vi "ini Read Key.vi"(0 "Refnum in":T1, 1 "Section":string, 2 "Key":string, 5 "Error In":errorcluster) -> (14 "Refnum out":T1, 15 "value":string, 19 "error out":errorcluster)   [LabVIEW 2016, in "Application.lvclass"]
uses:
  Application.lvclass
  <vilib>/Utility/config.llb/Config Data RefNum.ctl
  <vilib>/Utility/config.llb/Read Key (String).vi
  <vilib>/Utility/config.llb/NI_LVConfig.lvlib
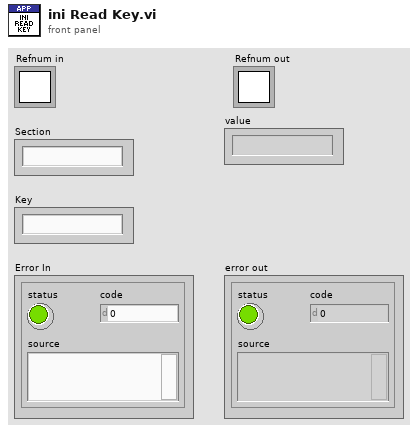
[diagram p1: front panel]
types:
  T1 = typedef "NI_LVConfig.lvlib/Config Data RefNum.ctl" = refnum<k1>
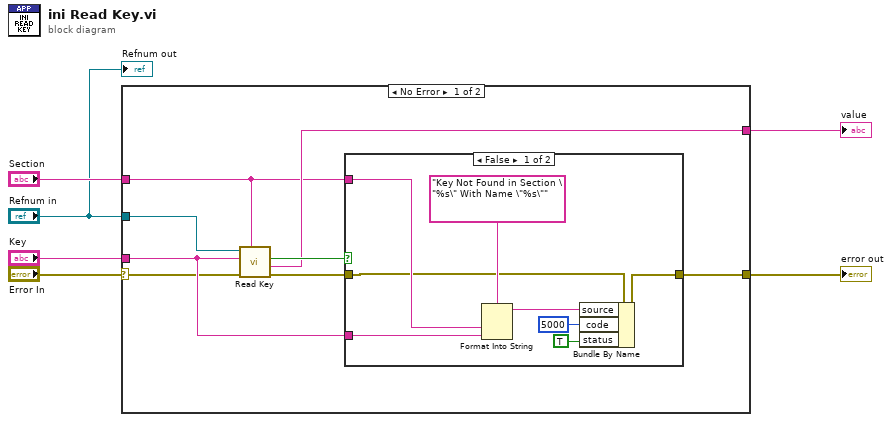
[diagram p0: block diagram]
diagram:
  n1 = case shown="No Error" "Error In" {
    selector: "Error In" -> [w7 w24]
    tunnel: [w14 w24] -> w6
    tunnel: [w11 _] -> w5
    tunnel: "Refnum in" -> [w10 _]
    tunnel: "Key" -> [w9 _]
    tunnel: "Section" -> [w8 _]
    frame No Error {
      n2 = call-poly <vilib>:"Read Key.vi"("section"=w8, "error in (no error)"=w7, "key"=w9, "refnum"=w10) -> ("error out"=w12:errorcluster, "value"=w11:string, "found?"=w13:bool)  [unwired: 4 in, 1 out]
      n3 = case shown="False" w13 {
        tunnel: w12 -> [w19 w23]
        tunnel: [w17 w23] -> w14
        tunnel: w9 -> [w21 _]
        tunnel: w8 -> [w22 _]
        frame False {
          n4 = Format Into String(format string="Key Not Found in Section \"%s\" With Name \"%s\"", w22, w21) -> (resulting string=w18:string)  [unwired: 2 in, 1 out]
          n5 = Bundle By Name(cluster=w19, "source"=w18, "code"=5000, "status"=TRUE) -> (w17:errorcluster)
        }
        frame True {
        }
      }
    }
    frame Error {
    }
  }
  "error out" <- w6
  "value" <- w5
  "Refnum out" <- "Refnum in"
